vi "ResponseHandler.vi"(11 "input string":string) -> (3 "x = y?":bool)   [LabVIEW 2017]
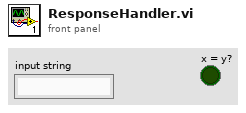
[diagram p1: front panel]
types:
  T1 = enum16{"EndOfLine", "LineFeed", "CarriageReturn"}
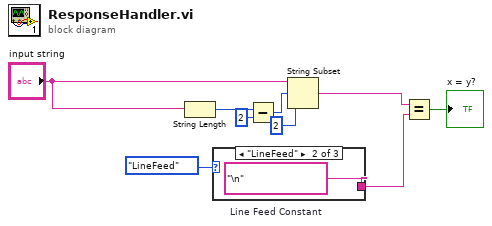
[diagram p0: block diagram]
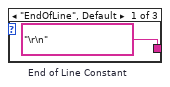
[diagram p2: hidden frame]
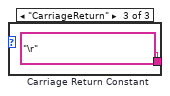
[diagram p3: hidden frame]
diagram:
  n1 = String Length(string="input string") -> (length=w5:i32)
  n2 = case shown="\"LineFeed\"" T1."LineFeed" {
    tunnel: [w10 w11 w12] -> w1
    frame "EndOfLine", Default {
      w10 = "\r\n"  # End of Line Constant
    }
    frame "LineFeed" {
      w11 = "\n"  # Line Feed Constant
    }
    frame "CarriageReturn" {
      w12 = "\r"  # Carriage Return Constant
    }
  }
  n3 = Subtract(x=w5, y=2) -> (x-y=w8:i32)
  n4 = String Subset(string="input string", offset (0)=w8, length (rest)=2 ("length (rest)")) -> (substring=w6:string)
  n5 = Equal?(x=w6, y=w1) -> (x = y?=→"x = y?":bool)
